vi "LogDBDoubleTimeArray.vi"(0 "Refnum in":T1, 1 "db Interval [s]":u32, 2 "db timing":i64, 3 "Actual Start [f] in":i64, 5 "db connection":bool, 7 "values":dbl[](array[numeric]), 11 "error in (no error)":errorcluster, 12 "Time Stamp":timestamp, 13 "prefix":string, 14 "names":string[](array[string])) -> (4 "Refnum out":T1, 6 "Actual Start [f] out":i64, 8 "db connection":bool, 15 "error out":errorcluster)   [LabVIEW 2011]
uses:
  <vilib>/addons/database/Connection.llb/Conn ObjectReference.ctl
  <vilib>/Utility/error.llb/DialogType.ctl
  <vilib>/addons/database/NI_Database_API.lvlib
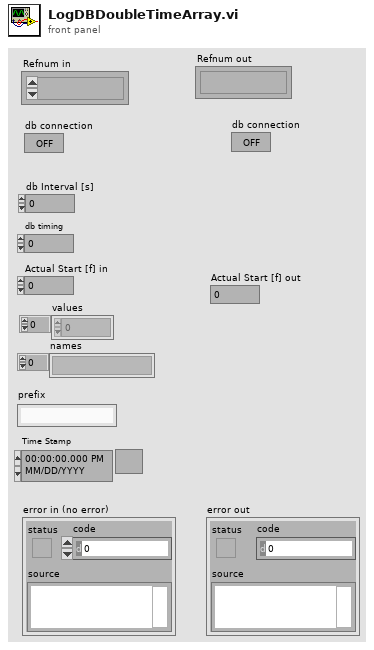
[diagram p1: front panel]
types:
  T1 = typedef "NI_Database_API.lvlib/Conn ObjectReference.ctl" = refnum<k1>
  T2 = typedef "DialogType.ctl" = u16
  T3 = cluster{"Time Stamp":timestamp, "pHS-1 [pH]":dbl}
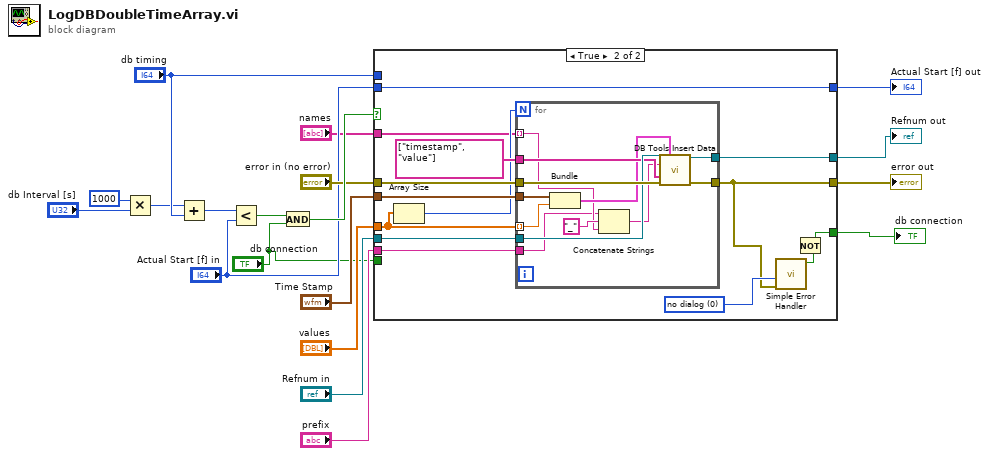
[diagram p0: block diagram]
diagram:
  n1 = Multiply(x=u32 1000, y="db Interval [s]") -> (x*y=w10:u32)
  n2 = Add(x=w10, y="db timing") -> (x+y=w8:i64)
  n3 = Less?(x=w8, y="Actual Start [f] in") -> (x < y?=w9:bool)
  n4 = And(x=w9, y="db connection") -> (x .and. y?=w19:bool)
  n5 = case shown="True" w19 {
    tunnel: [w23 w25] -> w16
    tunnel: "error in (no error)" -> [w23 w36]
    tunnel: [w22 w37] -> w14
    tunnel: "Actual Start [f] in" -> [_ w37]
    tunnel: "db timing" -> [w22 _]
    tunnel: "Refnum in" -> [w21 w35]
    tunnel: [w21 w30] -> w17
    tunnel: "Time Stamp" -> [_ w33]
    tunnel: "prefix" -> [_ w31]
    tunnel: "values" -> [_ w29]
    tunnel: "names" -> [_ w28]
    tunnel: [w20 w24] -> w1
    tunnel: "db connection" -> [w20 _]
    frame False {
    }
    frame True {
      w27 = T2 0 items=["no dialog", "OK message", "continue or stop message", "OK message + warnings", "continue/stop + warnings"] ("type of dialog (OK msg:1)")
      n6 = Array Size(array=w29) -> (size(s)=w32:i32)
      n7 = for {
        N: w32 -> [_]
        tunnel: w28 -> [w41] mode=indexing
        tunnel: [w38] -> w25
        tunnel: [w49] -> w30
        tunnel: w36 -> [w48]
        tunnel: w35 -> [w47]
        tunnel: string[] ["timestamp", "value"] ("columns") -> [w46]
        tunnel: w33 -> [w45]
        tunnel: w29 -> [w43] mode=indexing
        tunnel: w31 -> [w39]
        n8 = Bundle("Time Stamp"=w45, "pHS-1 [pH]"=w43) -> (w44:T3)  [unwired: 1 in]
        n9 = Concatenate Strings(w39, "_" ("string"), w41) -> (w40:string)
        n10 = call <vilib>:"DB Tools Insert Data.vi"("connection reference"=w47, "data"=w44, "table"=w40, "columns"=w46, "error in (no error)"=w48) -> ("connection reference out"=w49:T1, "error out"=w38:errorcluster)  [unwired: 9 in]
      }
      n11 = call <vilib>:"Simple Error Handler.vi"("type of dialog (OK msg:1)"=w27, "error in (no error)"=w25) -> ("error?"=w26:bool)  [unwired: 3 in, 4 out]
      n12 = Not(x=w26) -> (.not. x?=w24:bool)
    }
  }
  "Refnum out" <- w17
  "error out" <- w16
  "Actual Start [f] out" <- w14
  "db connection" <- w1
